vi "Deserialize Array.vi"(11 "Waypoints Array":T1) -> (3 "Serialized Waypoint Array":string[](array[string]))   [LabVIEW 2011]
doc: "Serializes an array of waypoints, producing an array of serialized waypoints.\nUsed for sending waypoints over a network, where sending object references does not work."
uses:
  0x2-OCU-Think Comm/0x2 Typedefs/Waypoints List.ctl
  Waypoint.lvclass
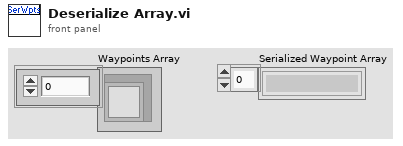
[diagram p1: front panel]
types:
  T1 = typedef "Waypoints List.ctl" = refnum<class "Waypoint.lvclass">[]
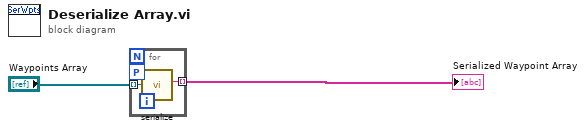
[diagram p0: block diagram]
diagram:
  n1 = for {
    tunnel: "Waypoints Array" -> [w4] mode=indexing
    tunnel: [w3] -> w2 mode=indexing
    workers-P: _ -> [_]
    n2 = call "serialize.vi"("Waypoint In"=w4) -> ("Flattened Waypoint"=w3:string)  [unwired: 9 in, 1 out]
  }
  "Serialized Waypoint Array" <- w2
